vi "F Dwf Analog Out Amplitude Get.vi"(8 "error in (no error)":errorcluster, 9 "pvoltsAmplitude":dbl, 10 "idxChannel":i32, 11 "hdwf":i32) -> (0 "error out":errorcluster, 1 "pvoltsAmplitude out":dbl, 3 "function return":i32)   [LabVIEW 2021, in "Olasdwf.lvlib"]
doc: "DWFAPI int FDwfAnalogOutAmplitudeGet(HDWF hdwf, int idxChannel, double *pvoltsAmplitude);"
uses:
  Olasdwf.lvlib
  Windows/System32/dwf.dll
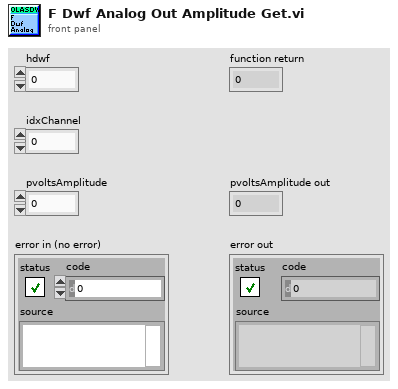
[diagram p1: front panel]
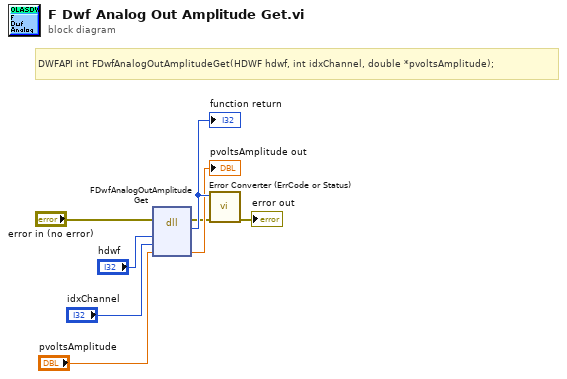
[diagram p0: block diagram]
diagram:
  # "DWFAPI int FDwfAnalogOutAmplitudeGet(HDWF hdwf, int idxChannel, double *pvoltsAmplitude);"
  n1 = dll-call lib="/Windows/System32/dwf.*" fn="FDwfAnalogOutAmplitudeGet"(error in="error in (no error)", "hdwf"="hdwf", "idxChannel"="idxChannel", "pvoltsAmplitude"="pvoltsAmplitude") -> (error out=w2:errorcluster, w8:i32, "pvoltsAmplitude"=→"pvoltsAmplitude out":dbl)  [unwired: 4 in, 1 out]
  "function return" <- w8
  n2 = call "Error Converter (ErrCode or Status).vi"("error in (no error)"=w2, "error code"=w8) -> ("error out"=→"error out":errorcluster)  [unwired: 9 in]
